vi "Check Limit&TestName Between STDF For Same Tester.vi"(8 "Test Name Array":string[](array[string]), 9 "Low Limit Array":dbl[](array[numeric]), 10 "High Limit Array":dbl[](array[numeric]), 11 "Result Length Array":i32[](array[numeric])) -> (0 "error out":errorcluster, 1 "Test Name":string, 2 "Low Limit":dbl, 3 "High Limit":dbl, 5 "Result Length":i32)   [LabVIEW 2018, in "STDF File Parser.lvclass"]
uses:
  STDF File Parser.lvclass
  <vilib>/Utility/error.llb/Error Cluster From Error Code.vi
  <vilib>/ErrorRing/Error Ring.xnode
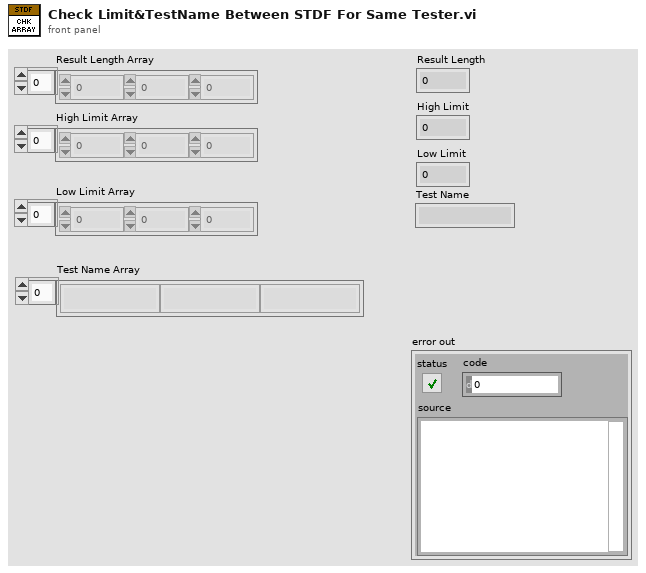
[diagram p1: front panel]
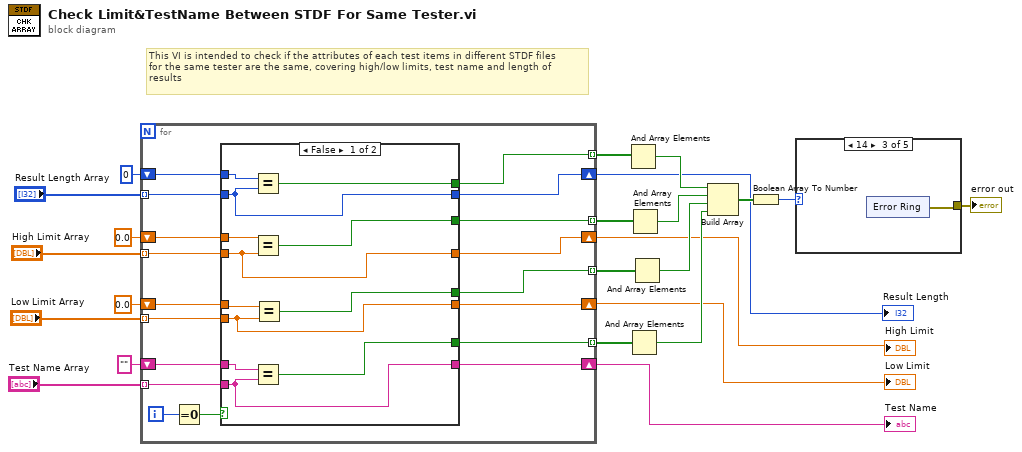
[diagram p0: block diagram]
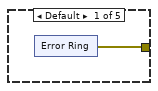
[diagram p2: hidden frame]
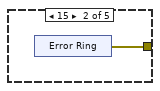
[diagram p3: hidden frame]
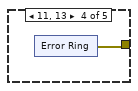
[diagram p4: hidden frame]
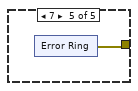
[diagram p5: hidden frame]
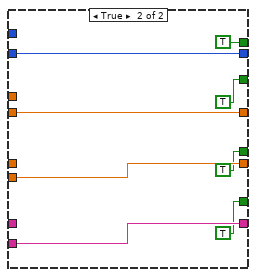
[diagram p6: hidden frame]
diagram:
  # "This VI is intended to check if the attributes of each test items in different STDF files\nfor the same tester are the same, covering high/low limits, test name and length of \nresults"
  n1 = for {
    tunnel: "High Limit Array" -> [w34] mode=indexing
    tunnel: "Low Limit Array" -> [w36] mode=indexing
    tunnel: "Test Name Array" -> [w39] mode=indexing
    shift-right: [w38] -> w2
    shift-left: "" ("String") -> [w37]
    shift-right: [w35] -> w3
    shift-left: 0.0 ("High Limit Array") -> [w31]
    shift-right: [w33] -> w4
    shift-left: 0.0 ("High Limit Array") -> [w32]
    tunnel: "Result Length Array" -> [w30] mode=indexing
    shift-right: [w29] -> w1
    shift-left: 0 ("High Limit Array") -> [w28]
    tunnel: [w27] -> w15 mode=indexing
    tunnel: [w26] -> w14 mode=indexing
    tunnel: [w25] -> w13 mode=indexing
    tunnel: [w24] -> w12 mode=indexing
    i -> [w41]
    n2 = Equal To 0?(x=w41) -> (x = 0?=w40:bool)
    n3 = case shown="False" w40 {
      tunnel: w39 -> [w46 w61]
      tunnel: [w46 w61] -> w38
      tunnel: w37 -> [w50 _]
      tunnel: w36 -> [w47 w60]
      tunnel: [w47 w60] -> w35
      tunnel: [w48 w59] -> w33
      tunnel: w34 -> [w48 w59]
      tunnel: w32 -> [w53 _]
      tunnel: w31 -> [w51 _]
      tunnel: w30 -> [w49 w58]
      tunnel: [w49 w58] -> w29
      tunnel: w28 -> [w52 _]
      tunnel: [w45 TRUE] -> w27
      tunnel: [w42 TRUE] -> w26
      tunnel: [w44 TRUE] -> w25
      tunnel: [w43 TRUE] -> w24
      frame False {
        n4 = Equal?(x=w52, y=w49) -> (x = y?=w45:bool)
        n5 = Equal?(x=w53, y=w48) -> (x = y?=w42:bool)
        n6 = Equal?(x=w50, y=w46) -> (x = y?=w43:bool)
        n7 = Equal?(x=w51, y=w47) -> (x = y?=w44:bool)
      }
      frame True {
      }
    }
  }
  "Test Name" <- w2
  "Low Limit" <- w3
  "High Limit" <- w4
  "Result Length" <- w1
  n8 = And Array Elements(Boolean array=w15) -> (logical AND=w11:bool)
  n9 = And Array Elements(Boolean array=w12) -> (logical AND=w8:bool)
  n10 = And Array Elements(Boolean array=w14) -> (logical AND=w10:bool)
  n11 = And Array Elements(Boolean array=w13) -> (logical AND=w9:bool)
  n12 = Build Array(w11, w10, w9, w8) -> (w7:bool[])
  n13 = Boolean Array To Number(Boolean array=w7) -> (number=w6:u32)
  n14 = case shown="14" w6 {
    tunnel: [w62 w68 w70 w76 w82] -> w5
    frame Default {
      n15 = xnode "Error Ring"() -> ("error out"=w62:errorcluster)
    }
    frame 15 {
      n16 = xnode "Error Ring"() -> ("error out"=w68:errorcluster)
    }
    frame 14 {
      n17 = xnode "Error Ring"() -> ("error out"=w70:errorcluster)
    }
    frame 11, 13 {
      n18 = xnode "Error Ring"() -> ("error out"=w76:errorcluster)
    }
    frame 7 {
      n19 = xnode "Error Ring"() -> ("error out"=w82:errorcluster)
    }
  }
  "error out" <- w5
